vi "PmacCoordStat.vi"(0 "Device Number i32 (0)":i32 min=0, 1 "Coord Number i32 (1-8) (1)":i32 min=0) -> (2 "First Word 24 Element Bool Array":bool[](array[boolean]), 3 "First Word Binary Status u32":u32 format="%.0x", 4 "Second Word 24 Element Bool Array":bool[](array[boolean]), 5 "Second Word Binary Status u32":u32 format="%.0x")   [LabVIEW 2020]
doc: "Query PMAC for the status of the CS specified by Coord Number. Report the two status words as arrays of booleans and unsigned 32 bit integers."
uses:
  Builds/5-8-13/data/PComm32W.dll
panel:
  # "Check the PMAC Documentation for Bit meanings!"
  # "Bit 23"
  # "Bit 0"
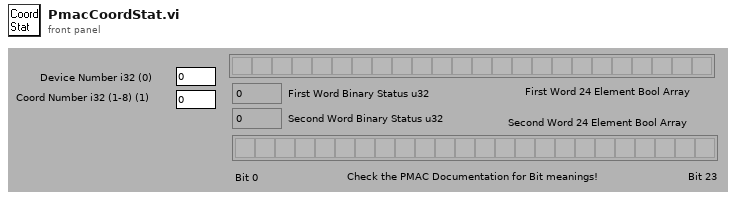
[diagram p1: front panel]
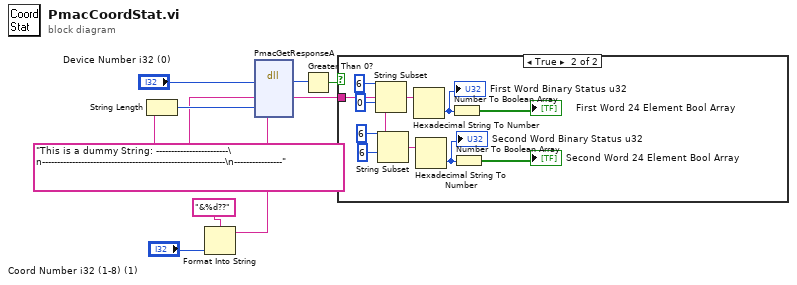
[diagram p0: block diagram]
diagram:
  w1 = "This is a dummy String: ------------------------\n-------------------------------------------------------------\n----------------"
  n1 = String Length(string=w1) -> (length=w8:i32)
  n2 = Format Into String(format string="&%d??", "Coord Number i32 (1-8) (1)") -> (resulting string=w5:string)  [unwired: 2 in, 1 out]
  n3 = dll-call lib="C:/NUWAR_Master/Builds/5-8-13/data/PComm32W.dll" fn="PmacGetResponseA"("DeviceNumber"="Device Number i32 (0)", "ResponseString"=w1, "MaxStringLength"=w8, "CommandString"=w5) -> (w4:i32, "ResponseString"=w2:string)  [unwired: 6 in, 2 out]
  n4 = Greater Than 0?(x=w4) -> (x > 0?=w3:bool)
  n5 = case shown="True" w3 {
    tunnel: w2 -> [_ w12]
    frame False {
    }
    frame True {
      n6 = String Subset(string=w12, offset (0)=0, length (rest)=6) -> (substring=w16:string)
      n7 = String Subset(string=w12, offset (0)=6, length (rest)=6) -> (substring=w20:string)
      n8 = Hexadecimal String To Number(string=w16) -> (number=w13:u32)  [unwired: 3 out]
      "First Word Binary Status u32" <- w13
      n9 = Hexadecimal String To Number(string=w20) -> (number=w17:u32)  [unwired: 3 out]
      "Second Word Binary Status u32" <- w17
      n10 = Number To Boolean Array(number=w13) -> (Boolean array=→"First Word 24 Element Bool Array":bool[])
      n11 = Number To Boolean Array(number=w17) -> (Boolean array=→"Second Word 24 Element Bool Array":bool[])
    }
  }
